vi "Do.vi"(8 "error in (no error)":errorcluster, 10 "Actor in":refnum<class "Actor.lvclass">, 11 "Class Loading Result Msg in":refnum<class "Class Loading Result Msg.lvclass">) -> (0 "error out":errorcluster, 2 "Actor out":refnum<class "Actor.lvclass">)   [LabVIEW 2023, in "Class Loader Interfaces.lvlib" / "Class Loading Result Msg.lvclass"]
doc: "This VI delivers the message to the actor by calling the appropriate method(s) on the actor."
uses:
  Class Loading Result Msg.lvclass
  Class Loading Result Msg.lvclass/Class Loading Result Msg.ctl
  e006e111-37be-4fe4-9230-d9ae1a3d60d7.vi
  Class Loader Interfaces/Class Loader Interfaces.lvclass
  <vilib>/ActorFramework/Actor/Actor.lvclass
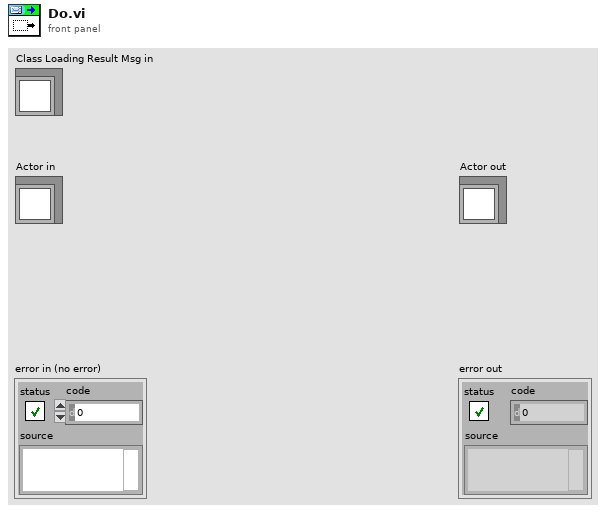
[diagram p1: front panel]
types:
  T1 = typedef "Class Loader.lvlib/Class Loader.lvclass/Classes Map.ctl" = map{string, refnum<class>}
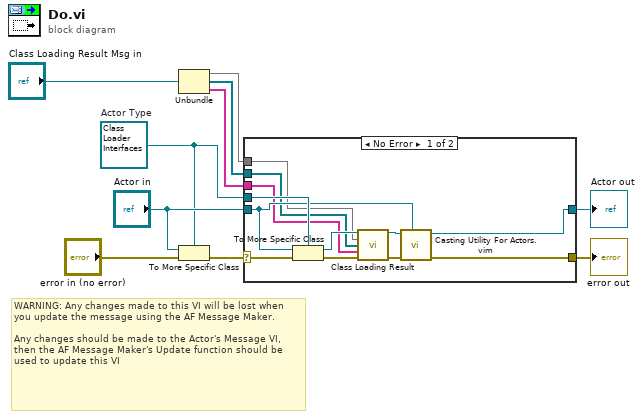
[diagram p0: block diagram]
diagram:
  w5 = refnum<class "Class Loader Interfaces.lvclass"> refnum  # Actor Type
  # "WARNING: Any changes made to this VI will be lost when you update the message using the AF Message Maker.\n\nAny changes should be made to the Actor's Message VI, then the AF Message Maker's Update function should be used to update this VI"
  n1 = Unbundle("Class Loading Result Msg in") -> (w4:T1, w3:refnum<class>[], w2:string[])
  n2 = To More Specific Class(target class=w5, reference="Actor in", error in="error in (no error)") -> (error out=w9:errorcluster)  [unwired: 1 out]
  n3 = case shown="No Error" w9 {
    selector: w9 -> [w18 w24]
    tunnel: [w20 w24] -> w8
    tunnel: [w19 w23] -> w7
    tunnel: "Actor in" -> [w21 w23]
    tunnel: w5 -> [w22 _]
    tunnel: w4 -> [w13 _]
    tunnel: w3 -> [w12 _]
    tunnel: w2 -> [w11 _]
    frame No Error {
      n4 = To More Specific Class ("Actor Cast")(target class=w22, reference=w21, error in=w18) -> (specific class reference=w17:refnum<class "Class Loader Interfaces.lvclass">, error out=w16:errorcluster)
      n5 = call-dynamic "Class Loading Result.vi"("Class Loader Interfaces in"=w17, "Classes Map"=w13, "Class Array"=w12, "Class Names"=w11, "error in (no error)"=w16) -> ("Class Loader Interfaces out"=w15:refnum<class "Class Loader Interfaces.lvclass">, "error out"=w14:errorcluster)  [unwired: 9 in]
      n6 = call "Casting Utility For Actors.vim"("type"=w21, "error in (no error)"=w14, "Actor in"=w15) -> ("error out"=w20:errorcluster, "Actor out"=w19:refnum<class "Actor.lvclass">)  [unwired: 7 in]
    }
    frame Error {
    }
  }
  "error out" <- w8
  "Actor out" <- w7
